vi "GetTTab.vi"(6 "错误输入（无错误）":errorcluster, 9 "Panel":refnum<vi>) -> (0 "错误输出":errorcluster, 3 "Pages":refnum<vi>[](array[refnum]))   [LabVIEW 2017]
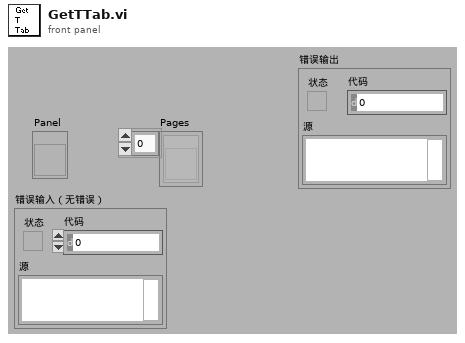
[diagram p1: front panel]
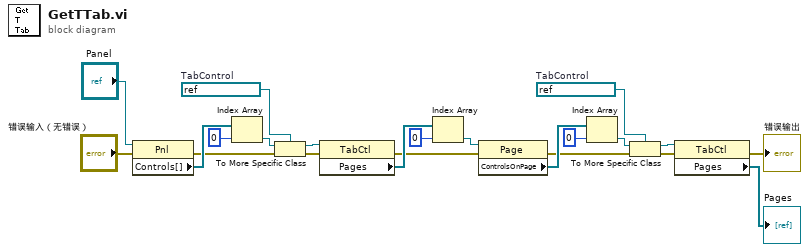
[diagram p0: block diagram]
diagram:
  w20 = refnum<vi> refnum  # TabControl
  w13 = refnum<vi> refnum  # TabControl
  n1 = property class="Pnl"(reference="Panel", error in="错误输入（无错误）") -> (error out=w7:errorcluster, "Controls[]"=w9:refnum<vi>[])  [unwired: 1 out]
  n2 = Index Array(array=w9, index=0 ("索引")) -> (element=w10:refnum<vi>)
  n3 = To More Specific Class(target class=w13, reference=w10, error in=w7) -> (specific class reference=w11:refnum<vi>, error out=w6:errorcluster)
  n4 = property class="TabCtl"(reference=w11, error in=w6) -> (error out=w5:errorcluster, "Pages"=w12:refnum<vi>[])  [unwired: 1 out]
  n5 = Index Array(array=w12, index=0 ("索引")) -> (element=w16:refnum<vi>)
  n6 = property class="Page"(reference=w16, error in=w5) -> (error out=w4:errorcluster, "ControlsOnPage"=w22:refnum<vi>[])  [unwired: 1 out]
  n7 = Index Array(array=w22, index=0 ("索引")) -> (element=w21:refnum<vi>)
  n8 = To More Specific Class(target class=w20, reference=w21, error in=w4) -> (specific class reference=w18:refnum<vi>, error out=w3:errorcluster)
  n9 = property class="TabCtl"(reference=w18, error in=w3) -> (error out=→"错误输出":errorcluster, "Pages"=→"Pages":refnum<vi>[])  [unwired: 1 out]
